vi "Drivetrain Log Write.vi"(8 "drive log":refnum<file>, 9 "Drive Cmd Packet":T1) -> ()   [LabVIEW 2014]
uses:
  TeleopCmd.ctl
  CmdFlag.ctl
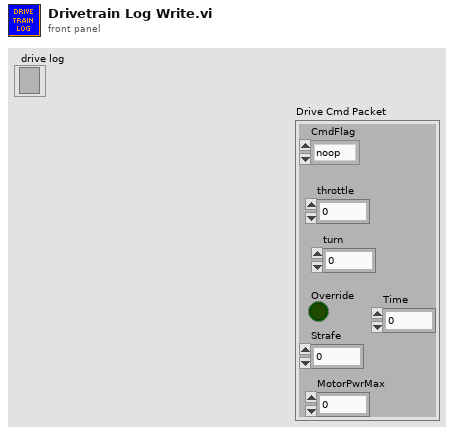
[diagram p1: front panel]
types:
  T1 = typedef "TeleopCmd.ctl" = cluster{"CmdFlag":T2, "throttle":dbl, "turn":dbl, "Override":bool, "Strafe":dbl, "MotorPwrMax":u8, "Time":u32}
  T2 = typedef "CmdFlag.ctl" = enum16{"noop", "suspend", "resume"}
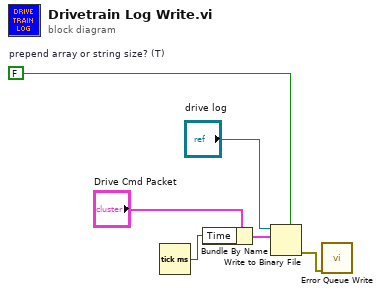
[diagram p0: block diagram]
diagram:
  w2 = FALSE  # prepend array or string size? (T)
  n1 = Tick Count (ms)() -> (millisecond timer value=w5:u32)
  n2 = Bundle By Name(cluster="Drive Cmd Packet", "Time"=w5) -> (w4:T1)
  n3 = Write to Binary File(file (use dialog)="drive log", data=w4, 5:w2) -> (error out=w1:errorcluster)  [unwired: 3 in, 2 out]
  n4 = call "Error Queue Write.vi"("error in (no error)"=w1) -> ()  [unwired: 11 in]
